vi "Find Fiducial.vi"(4 "Image":T2(plugin-control)) -> (0 "Move by (mm)":dbl[](array[numeric]) format="%#_9g")   [LabVIEW 2020]
panel:
  out "Current":dbl[](array[numeric])
  out "Center":dbl[](array[numeric])
  out "Results":T1(array[cluster]) {"Score" format="%.1f"; "Position"."Y" format="%.3g"; "Position"."X" format="%.3g"}
  out "Template":T2(plugin-control)
  in  "image path":path=path "C:/Users/HEP/Documents/Aerotech gantry/Sindhu/Pattern recog/ref2.png"
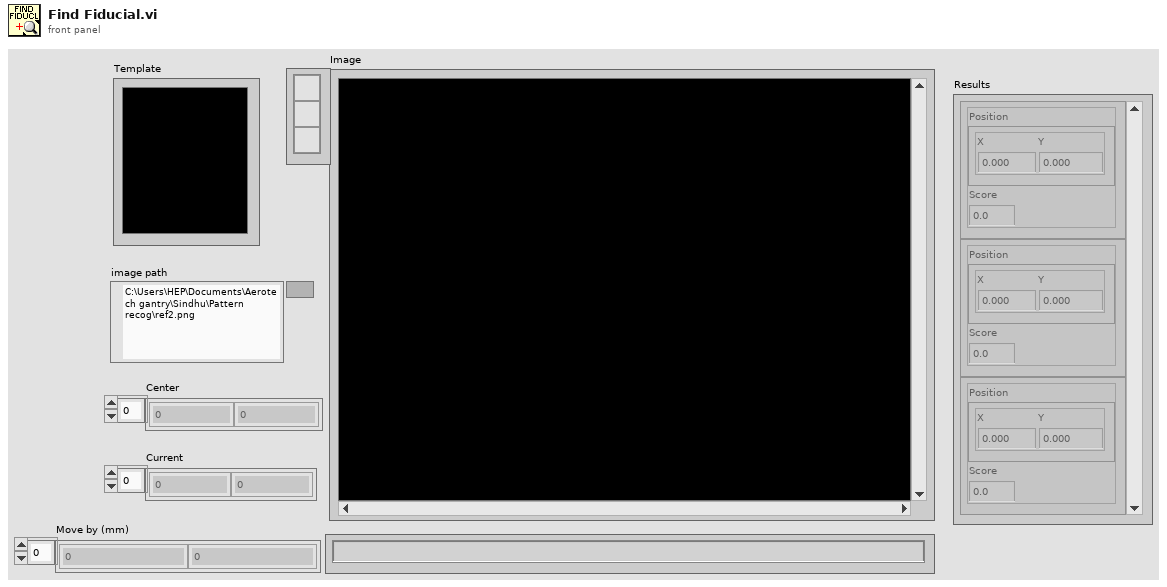
[diagram p1: front panel]
types:
  T1 = cluster{"Position":cluster{"X":dbl, "Y":dbl}, "Score":sgl}[]
  T2 = typedef "IMAQ Image.ctl" = refnum<image>
  T3 = cluster{"Position":cluster{"X":dbl, "Y":dbl}, "Score":sgl}
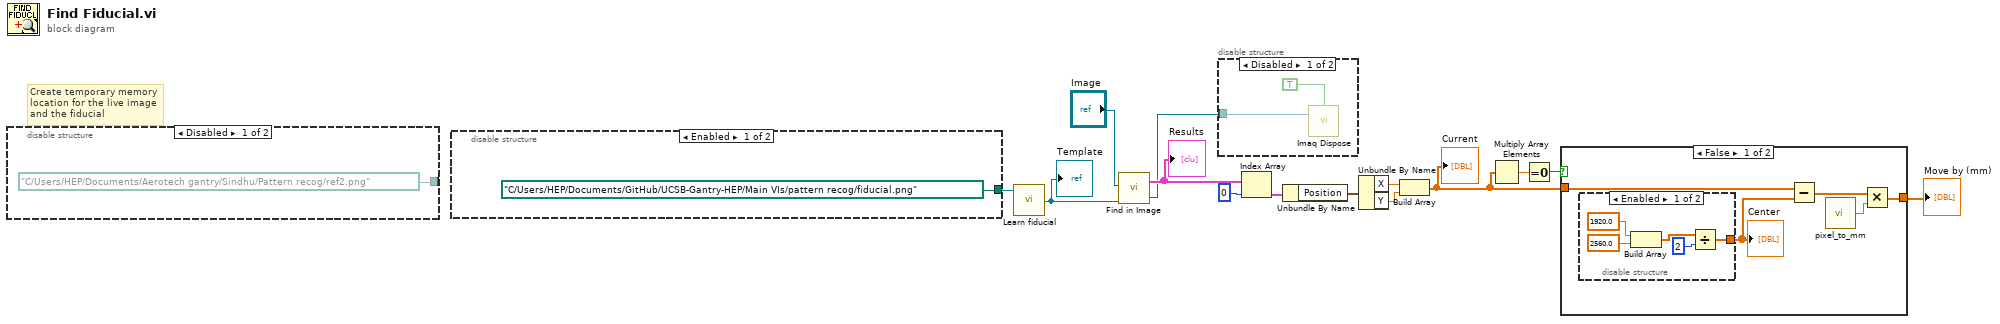
[diagram p0: block diagram]
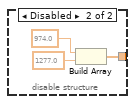
[diagram p3: hidden frame]
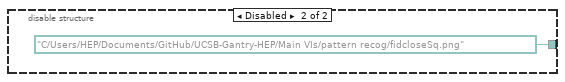
[diagram p5: hidden frame]
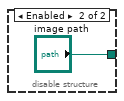
[diagram p6: hidden frame]
diagram:
  # "Create temporary memory location for the live image and the fiducial"
  n1 = disable-structure shown="Disabled" {
    disable-tunnel: [path "C:/Users/HEP/Documents/Aerotech gantry/Sindhu/Pattern recog/ref2.png" ("name or relative path") "image path"] -> _
    frame Disabled {
    }
    frame Enabled {
    }
  }
  n2 = disable-structure shown="Enabled" {
    disable-tunnel: [path "C:/Users/HEP/Documents/GitHub/UCSB-Gantry-HEP/Main VIs/pattern recog/fiducial.png" ("name or relative path") path "C:/Users/HEP/Documents/GitHub/UCSB-Gantry-HEP/Main VIs/pattern recog/fidcloseSq.png" ("name or relative path")] -> w14
    frame Enabled {
    }
    frame Disabled {
    }
  }
  n3 = call "Learn fiducial.vi"("template path"=w14) -> ("Template"=w7:T2)  [unwired: 1 in]
  "Template" <- w7
  n4 = call "Find in Image.vi"("Template"=w7, "Image"="Image") -> ("Image Out"=w1:T2, "Results"=w8:T1)  [unwired: 2 in]
  "Results" <- w8
  n5 = disable-structure shown="Disabled" {
    disable-tunnel: w1 -> [w20 _]
    frame Disabled {
      n6 = call "Imaq Dispose"("All Images? (No)"=TRUE, "Image"=w20) -> ()  [unwired: 4 in, 1 out]
    }
    frame Enabled {
    }
  }
  n7 = Index Array(array=w8, index=0) -> (element=w12:T3)
  n8 = Unbundle By Name(w12) -> ("Position"=w11:cluster{"X":dbl, "Y":dbl})
  n9 = Unbundle By Name(w11) -> ("X"=w10:dbl, "Y"=w9:dbl)
  n10 = Build Array(w10, w9) -> (w2:dbl[])
  "Current" <- w2
  n11 = Multiply Array Elements(1:w2) -> (0:w4:dbl)
  n12 = Equal To 0?(x=w4) -> (x = 0?=w3:bool)
  n13 = case shown="False" w3 {
    tunnel: w2 -> [w25 w34]
    tunnel: [w21 w34] -> w5
    frame False {
      n14 = disable-structure shown="Enabled" {
        disable-tunnel: [w26 w31] -> w24
        frame Enabled {
          n15 = Build Array(1920.0, 2560.0) -> (w28:dbl[])
          n16 = Divide(x=w28, y=2) -> (x/y=w26:dbl[])
        }
        frame Disabled {
          n17 = Build Array(974.0, 1277.0) -> (w31:dbl[])
        }
      }
      "Center" <- w24
      n18 = Subtract(x=w25, y=w24) -> (x-y=w23:dbl[])
      n19 = call "pixel_to_mm.vi"() -> ("mm/pixel"=w22:dbl)  [unwired: 2 in]
      n20 = Multiply(x=w23, y=w22) -> (x*y=w21:dbl[])
    }
    frame True {
    }
  }
  "Move by (mm)" <- w5
